vi "6-18-19 Increasing Temp.vi"() -> ()   [LabVIEW 2016]
uses:
  <vilib>/Analysis/baseanly.llb/Mean (DBL).vi
  <userlib>/Levylab/LV to ITX/LVtoITX.lvclass
  <vilib>/Analysis/NI_AALBase.lvlib
  <vilib>/Analysis/NI_AALPro.lvlib
panel:
  out "dG/dt/G":cluster{dbl[], "Best Exponential Fit":dbl[]}[](graph)
  out "G v T, norm vs prev":cluster{dbl[], "Best Exponential Fit":dbl[]}[](graph)
  out "G v T, norm vs 275":cluster{dbl[], "Best Exponential Fit":dbl[]}[](graph)
  in  "Path":path=path "G:/My Drive/Data/6-18 Increasing SA40060.dat"
  out "output cluster":cluster{dbl[], dbl[], dbl[], dbl[]}
  out "Temp vs Time":cluster{dbl[], dbl[]}(graph)
  out "Time vs Temp":cluster{dbl[], dbl[]}(graph)
  out "G4T Vs Temp":cluster{"Data":dbl[], "Data":dbl[]}[](graph)
  out "G2T Vs Temp":cluster{"Data":dbl[], "Data":dbl[]}[](graph)
  out "Linear Fit":cluster{dbl[], "Best Exponential Fit":dbl[]}[](graph)
  out "Full Data":cluster{dbl[], dbl[]}[](graph)
  in  "header length":i32=37
  out "Comments":string
  out "Wavenames":string[](array[string])
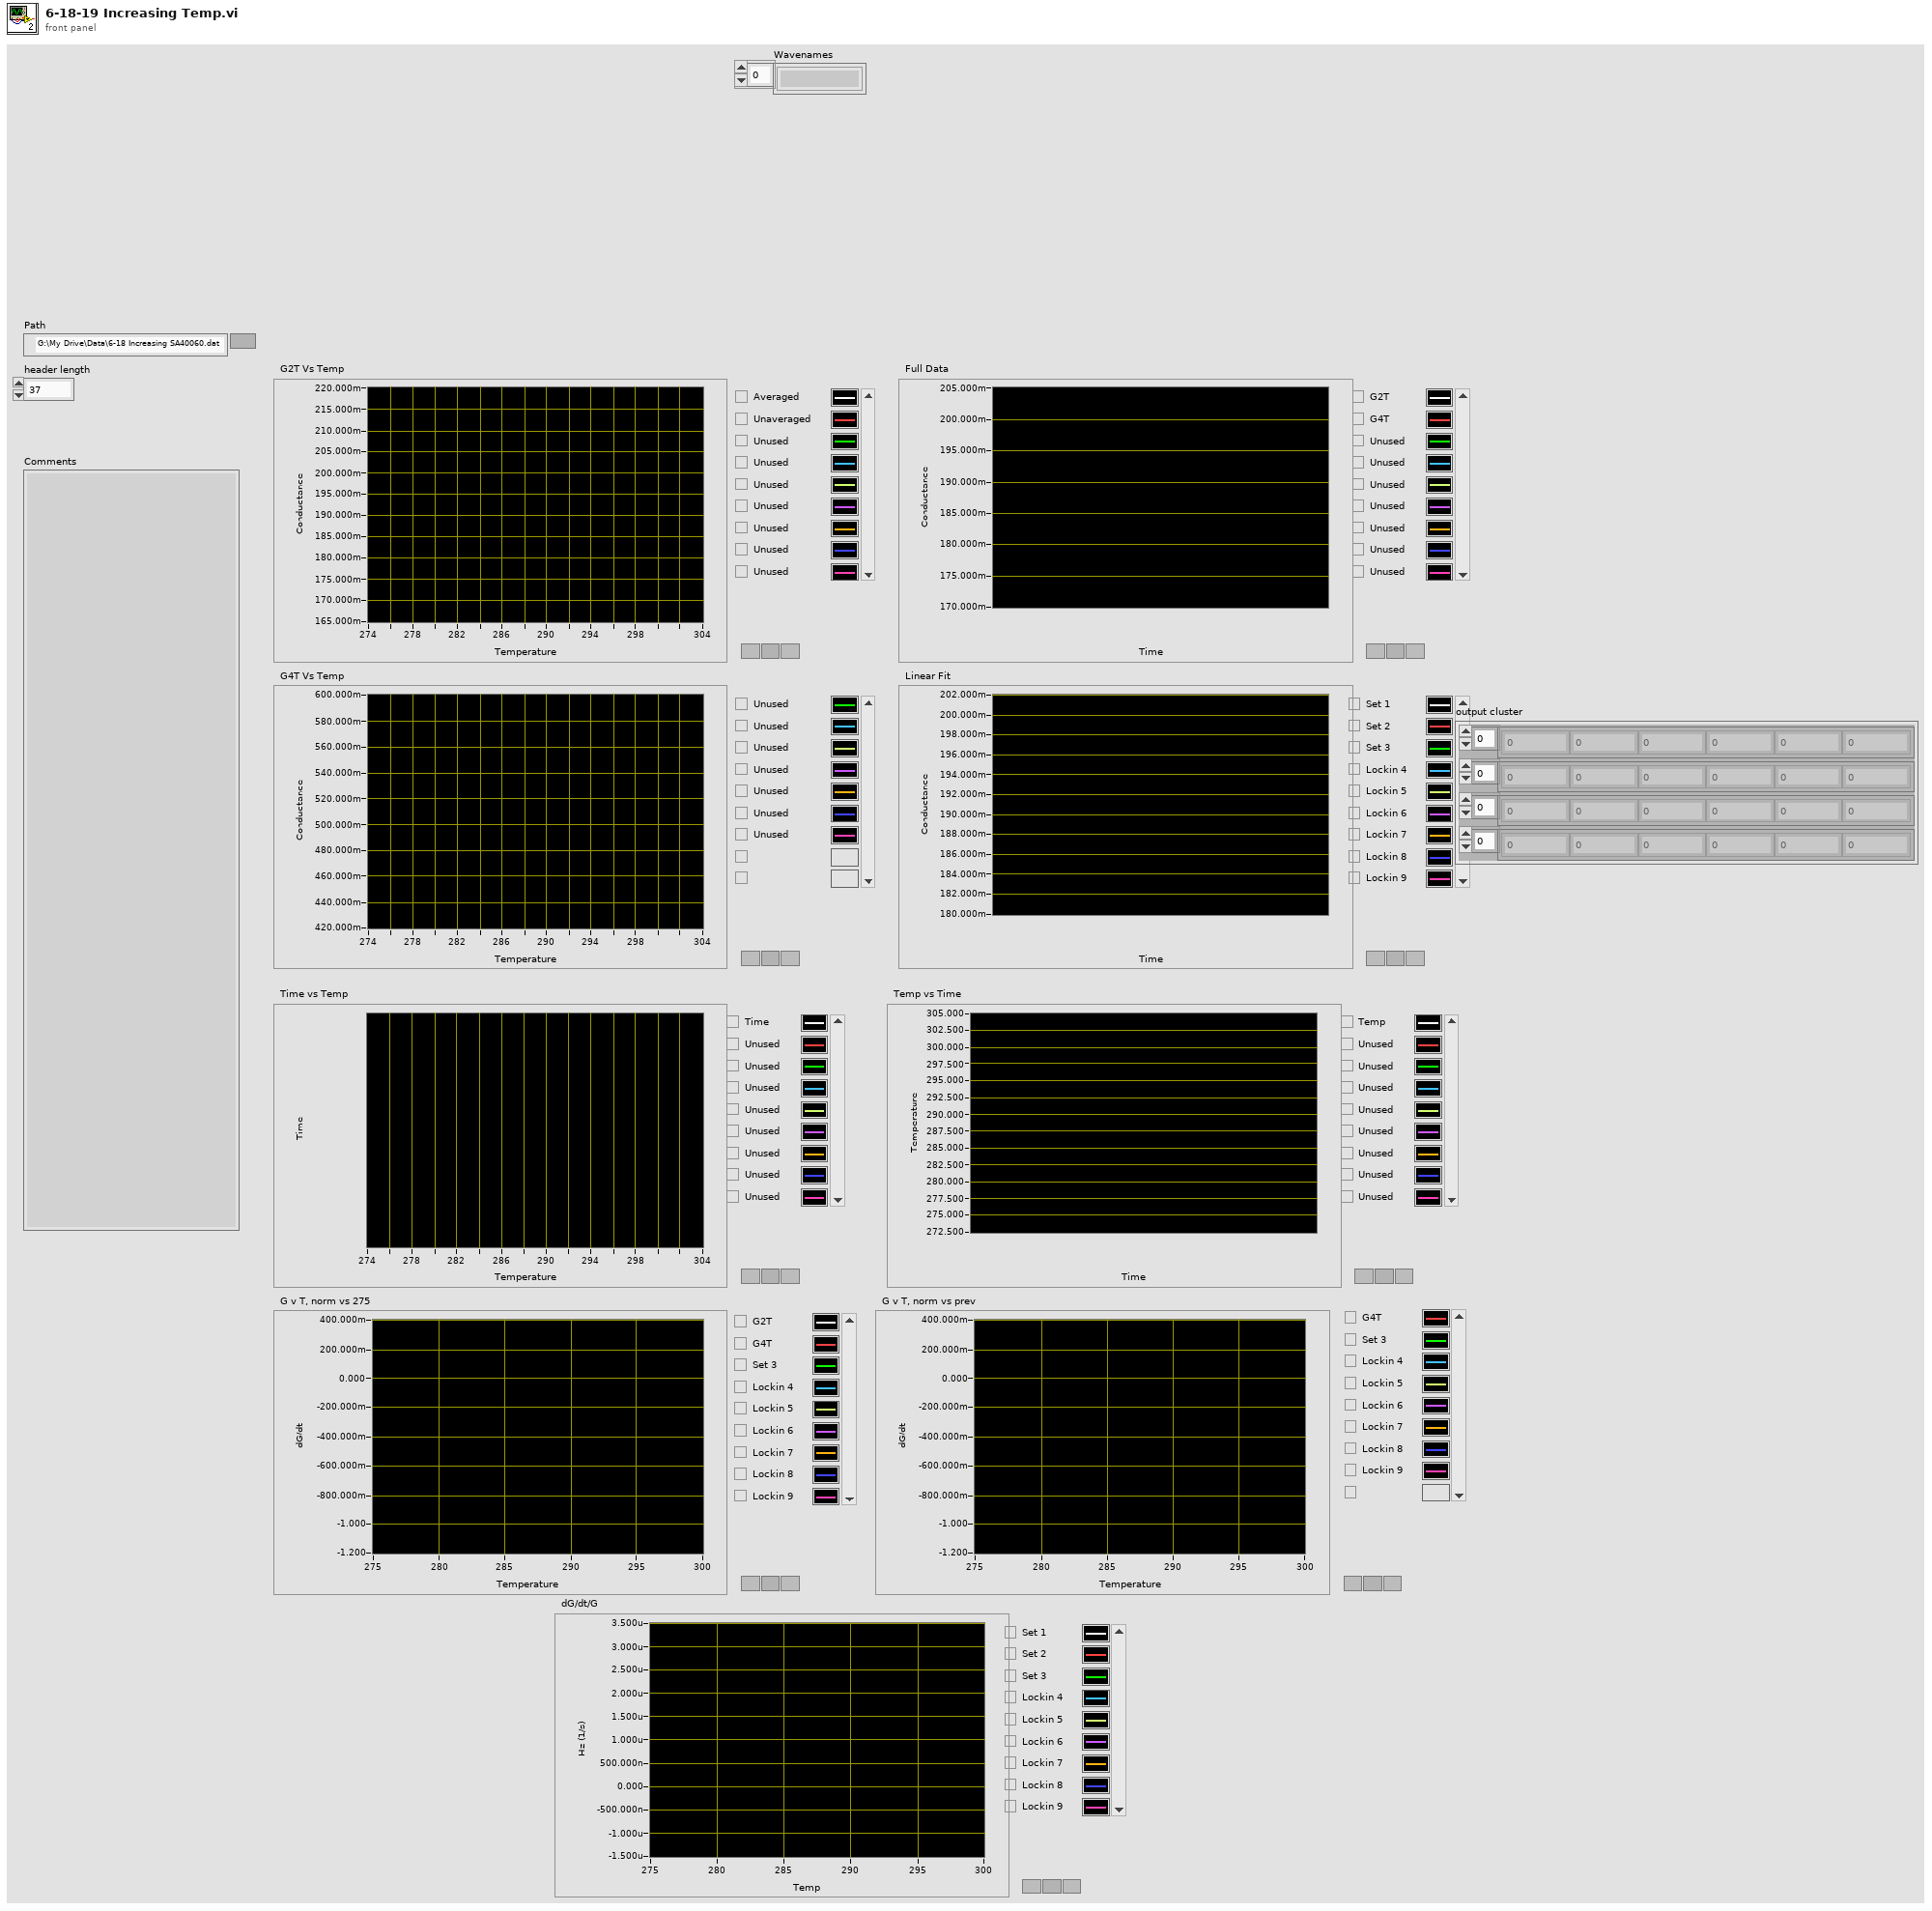
[diagram p1: front panel]
types:
  T1 = cluster{"slope min":dbl, "slope max":dbl, "intercept min":dbl, "intercept max":dbl}
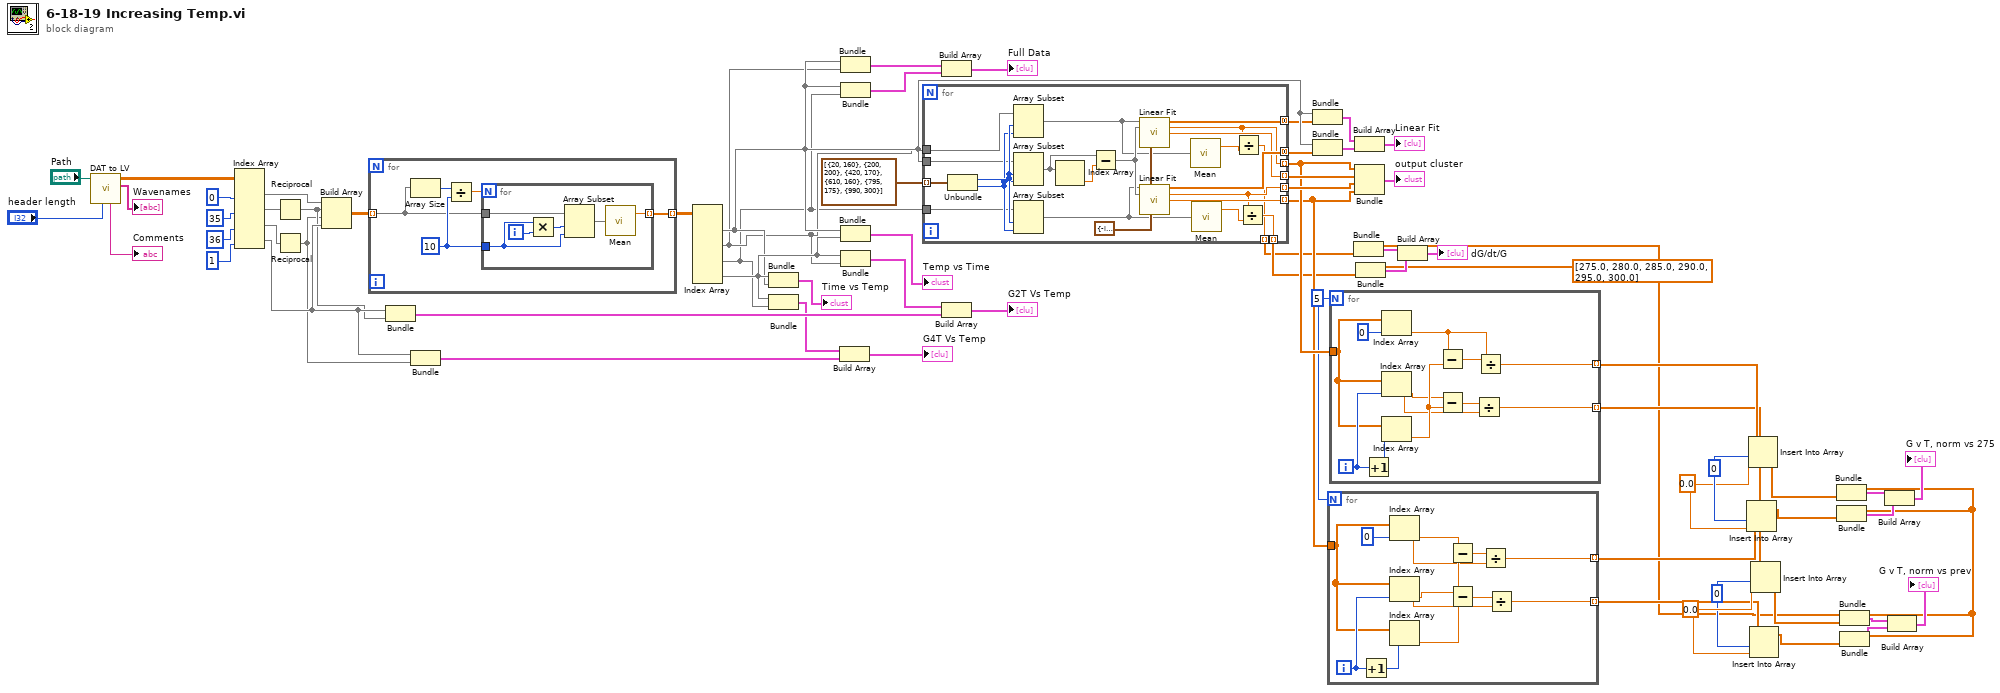
[diagram p0: block diagram]
diagram:
  w11 = 5
  w21 = 0.0
  w20 = 0
  w3 = dbl[] [275.0, 280.0, 285.0, 290.0, 295.0, 300.0]
  w26 = 0.0
  w27 = 0
  n1 = call <userlib>:"DAT to LV.vi"("header length"="header length", "File Path"="Path") -> ("Wavenames"=→"Wavenames":string[], "Data"=w66:dbl[][], "Comments"=→"Comments":string)  [unwired: 6 in, 1 out]
  n2 = Index Array(array=w66, index (col) #1=0 ("disabled index (col)"), index (col) #2=35 ("index (col)"), index (col) #3=36 ("index (col)"), index (col) #4=1 ("index (col)")) -> (element #1=w37:dbl[], element #2=w33:dbl[], element #3=w31:dbl[], element #4=w36:dbl[])  [unwired: 4 in]
  n3 = Reciprocal(x=w33) -> (1/x=w32:dbl[])
  n4 = Reciprocal(x=w31) -> (1/x=w30:dbl[])
  n5 = Build Array(w37, w32, w30, w36) -> (w62:dbl[][])
  n6 = for {
    tunnel: w62 -> [w70] mode=indexing
    tunnel: [w69] -> w61 mode=indexing
    w71 = 10 ("x")
    n7 = Array Size(array=w70) -> (size(s)=w73:i32)
    n8 = Divide(x=w73, y=w71) -> (x/y=w72:dbl)
    n9 = for {
      N: w72 -> [_]
      tunnel: w71 -> [w77]
      tunnel: [w76] -> w69 mode=indexing
      tunnel: w70 -> [w75]
      i -> [w79]
      n10 = Multiply(x=w77, y=w79) -> (x*y=w78:i32)
      n11 = Array Subset(array=w75, index=w78, length=w77) -> (w74:dbl[])
      n12 = call-poly <vilib>:"Mean.vi"("X"=w74) -> ("mean"=w76:dbl)  [unwired: 1 out]
    }
  }
  n13 = Bundle("Data"=w36, w32) -> (w49:cluster{"Data":dbl[], dbl[]})  [unwired: 1 in]
  n14 = Bundle("Data"=w36, w30) -> (w48:cluster{"Data":dbl[], dbl[]})  [unwired: 1 in]
  n15 = Index Array(array=w61) -> (element #1=w42:dbl[], element #2=w40:dbl[], element #3=w39:dbl[], element #4=w68:dbl[])  [unwired: 8 in]
  n16 = Bundle(w68, w42) -> (→"Time vs Temp":cluster{dbl[], dbl[]})  [unwired: 1 in]
  n17 = Bundle(w68, w39) -> (w47:cluster{dbl[], dbl[]})  [unwired: 1 in]
  n18 = Build Array(w47, w48) -> (→"G4T Vs Temp":cluster{"Data":dbl[], dbl[]}[])
  n19 = Bundle(w42, w40) -> (w60:cluster{dbl[], dbl[]})  [unwired: 1 in]
  n20 = Bundle(w42, w39) -> (w59:cluster{dbl[], dbl[]})  [unwired: 1 in]
  n21 = Bundle(w42, w68) -> (→"Temp vs Time":cluster{dbl[], dbl[]})  [unwired: 1 in]
  n22 = Bundle(w68, w40) -> (w46:cluster{dbl[], dbl[]})  [unwired: 1 in]
  n23 = for {
    tunnel: cluster{i32, i32}[] [{20, 160}, {200, 200}, {420, 170}, {610, 160}, {795, 175}, {990, 300}] -> [w101] mode=indexing
    tunnel: w42 -> [w98]
    tunnel: w40 -> [w97]
    tunnel: w39 -> [w96]
    tunnel: [w95] -> w29 mode=concatenating
    tunnel: [w94] -> w28 mode=concatenating
    tunnel: [w85] -> w13 mode=indexing
    tunnel: [w90] -> w51 mode=indexing
    tunnel: [w82] -> w35 mode=indexing
    tunnel: [w89] -> w12 mode=indexing
    tunnel: [w81] -> w2 mode=indexing
    tunnel: [w80] -> w1 mode=indexing
    w88 = T1 {"slope min"=-inf, "slope max"=inf, "intercept min"=-inf, "intercept max"=inf} ("parameter bounds")
    n24 = Unbundle(w101) -> (w100:i32, w99:i32)
    n25 = Array Subset(array=w97, index=w100, length=w99) -> (w86:dbl[])
    n26 = Array Subset(array=w98, index=w100, length=w99) -> (w93:dbl[])
    n27 = Array Subset(array=w96, index=w100, length=w99) -> (w87:dbl[])
    n28 = Index Array(array=w93) -> (element=w92:dbl)  [unwired: 1 in]
    n29 = Subtract(x=w93, y=w92) -> (x-y=w91:dbl[])
    n30 = call <vilib>:"Linear Fit.vi"("Y"=w86, "X"=w91, "parameter bounds"=w88) -> ("Best Linear Fit"=w95:dbl[], "slope"=w85:dbl, "intercept"=w90:dbl)  [unwired: 8 in, 2 out]
    n31 = call <vilib>:"Linear Fit.vi"("Y"=w87, "X"=w91, "parameter bounds"=w88) -> ("Best Linear Fit"=w94:dbl[], "slope"=w82:dbl, "intercept"=w89:dbl)  [unwired: 8 in, 2 out]
    n32 = call-poly <vilib>:"Mean.vi"("X"=w86) -> ("mean"=w84:dbl)  [unwired: 1 out]
    n33 = call-poly <vilib>:"Mean.vi"("X"=w87) -> ("mean"=w83:dbl)  [unwired: 1 out]
    n34 = Divide(x=w85, y=w84) -> (x/y=w80:dbl)
    n35 = Divide(x=w82, y=w83) -> (x/y=w81:dbl)
  }
  n36 = Build Array(w60, w59) -> (→"Full Data":cluster{dbl[], dbl[]}[])
  n37 = Build Array(w46, w49) -> (→"G2T Vs Temp":cluster{"Data":dbl[], dbl[]}[])
  n38 = Bundle(w42, "Best Linear Fit"=w29) -> (w53:cluster{dbl[], "Best Linear Fit":dbl[]})  [unwired: 1 in]
  n39 = Bundle(w42, "Best Linear Fit"=w28) -> (w52:cluster{dbl[], "Best Linear Fit":dbl[]})  [unwired: 1 in]
  n40 = for {
    N: w11 -> [_]
    tunnel: w12 -> [w109]
    tunnel: [w104] -> w7 mode=indexing
    tunnel: [w102] -> w8 mode=indexing
    i -> [w110]
    n41 = Increment(x=w110) -> (x+1=w111:i32)
    n42 = Index Array(array=w109, index=0) -> (element=w103:dbl)
    n43 = Index Array(array=w109, index=w110) -> (element=w105:dbl)
    n44 = Index Array(array=w109, index=w111) -> (element=w108:dbl)
    n45 = Subtract(x=w103, y=w108) -> (x-y=w107:dbl)
    n46 = Subtract(x=w105, y=w108) -> (x-y=w106:dbl)
    n47 = Divide(x=w107, y=w103) -> (x/y=w102:dbl)
    n48 = Divide(x=w106, y=w105) -> (x/y=w104:dbl)
  }
  n49 = for {
    N: w11 -> [_]
    tunnel: w13 -> [w120]
    tunnel: [w116] -> w10 mode=indexing
    tunnel: [w113] -> w9 mode=indexing
    i -> [w121]
    n50 = Increment(x=w121) -> (x+1=w122:i32)
    n51 = Index Array(array=w120, index=0) -> (element=w118:dbl)
    n52 = Index Array(array=w120, index=w121) -> (element=w114:dbl)
    n53 = Index Array(array=w120, index=w122) -> (element=w119:dbl)
    n54 = Subtract(x=w118, y=w119) -> (x-y=w117:dbl)
    n55 = Subtract(x=w114, y=w119) -> (x-y=w115:dbl)
    n56 = Divide(x=w115, y=w114) -> (x/y=w113:dbl)
    n57 = Divide(x=w117, y=w118) -> (x/y=w116:dbl)
  }
  n58 = Bundle(w3, w1) -> (w4:cluster{dbl[], dbl[]})  [unwired: 1 in]
  n59 = Build Array(w53, w52) -> (→"Linear Fit":cluster{dbl[], "Best Linear Fit":dbl[]}[])
  n60 = Bundle(w13, w51, w35, w12) -> (→"output cluster":cluster{dbl[], dbl[], dbl[], dbl[]})  [unwired: 1 in]
  n61 = Bundle(w3, w2) -> (w5:cluster{dbl[], dbl[]})  [unwired: 1 in]
  n62 = Build Array(w4, w5) -> (→"dG/dt/G":cluster{dbl[], dbl[]}[])
  n63 = Insert Into Array(array=w8, index=w27, new element=w26) -> (w25:dbl[])
  n64 = Insert Into Array(array=w10, index=w27, new element=w26) -> (w24:dbl[])
  n65 = Insert Into Array(array=w7, index=w20, new element=w21) -> (w18:dbl[])
  n66 = Insert Into Array(array=w9, index=w20, new element=w21) -> (w19:dbl[])
  n67 = Bundle(w3, w24) -> (w23:cluster{dbl[], dbl[]})  [unwired: 1 in]
  n68 = Bundle(w3, w25) -> (w22:cluster{dbl[], dbl[]})  [unwired: 1 in]
  n69 = Bundle(w3, w19) -> (w17:cluster{dbl[], dbl[]})  [unwired: 1 in]
  n70 = Bundle(w3, w18) -> (w16:cluster{dbl[], dbl[]})  [unwired: 1 in]
  n71 = Build Array(w23, w22) -> (→"G v T, norm vs 275":cluster{dbl[], dbl[]}[])
  n72 = Build Array(w17, w16) -> (→"G v T, norm vs prev":cluster{dbl[], dbl[]}[])
